vi "MouseMoveSingleY.vi"(10 "Delta":i32, 11 "XYGraph输入":refnum<vi>) -> ()   [LabVIEW 2015]
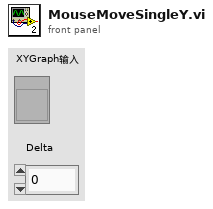
[diagram p1: front panel]
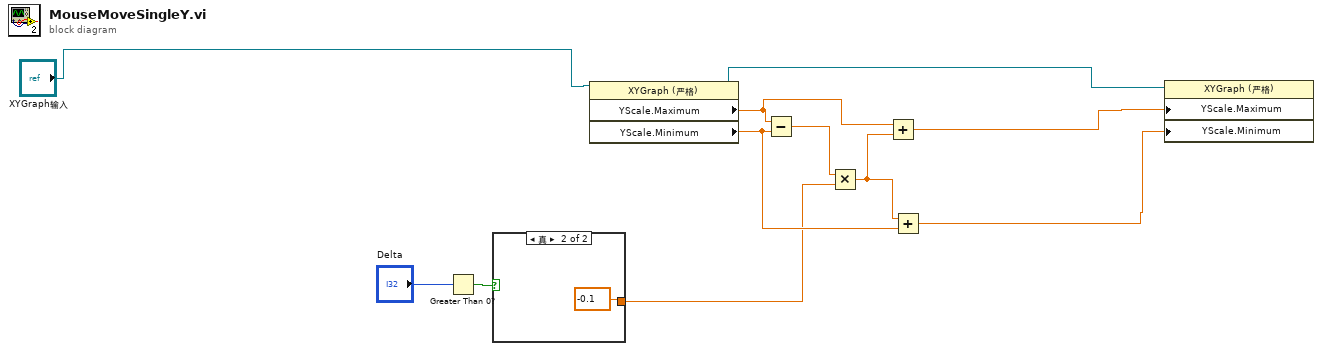
[diagram p0: block diagram]
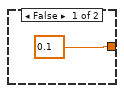
[diagram p2: hidden frame]
diagram:
  n1 = Greater Than 0?(x="Delta") -> (x > 0?=w11:bool)
  n2 = case shown="真" w11 {
    tunnel: [0.1 -0.1] -> w1
    frame False {
    }
    frame True {
    }
  }
  n3 = property class="XYGraph (严格)"(reference="XYGraph输入") -> (reference out=w9:refnum<vi>, "YScale.Maximum"=w6:dbl, "YScale.Minimum"=w4:dbl)  [unwired: 1 in, 1 out]
  n4 = Subtract(x=w6, y=w4) -> (x-y=w7:dbl)
  n5 = Multiply(x=w7, y=w1) -> (x*y=w5:dbl)
  n6 = Add(x=w6, y=w5) -> (x+y=w3:dbl)
  n7 = Add(x=w5, y=w4) -> (x+y=w2:dbl)
  n8 = property class="XYGraph (严格)"(reference=w9, "YScale.Maximum"=w3, "YScale.Minimum"=w2) -> ()  [unwired: 1 in, 2 out]
